vi "Config Voltage.vi"(0 "VISA resource name":refnum<visa-resource-name>, 1 "Element (0: All)":u16(ring) items=["All", "Element 1", "Element 2", "Element 3", "Element 4"], 7 "V Range (8: 2000)":u16(ring)=8 items=["AUTO", "30", "60", "120", "200", "300", "600", "1200", "2000"], 11 "error in (no error)":errorcluster) -> (4 "VISA resource name out":refnum<visa-resource-name>, 15 "error out":errorcluster)   [LabVIEW 2013, in "Yokogawa PZ4000.lvlib"]
doc: "This VI sends the Voltage Configure command to the PZ4000 series.\nConfigure Control Functions are Selects the Voltage Mode, Voltage Range and Element."
uses:
  <instrlib>/Yokogawa PZ4000/Yokogawa PZ4000.lvlib
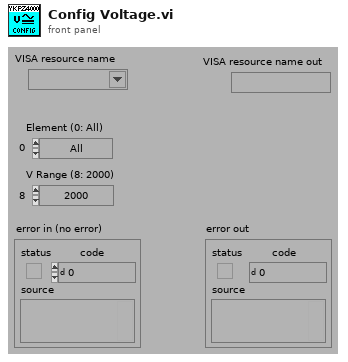
[diagram p1: front panel]
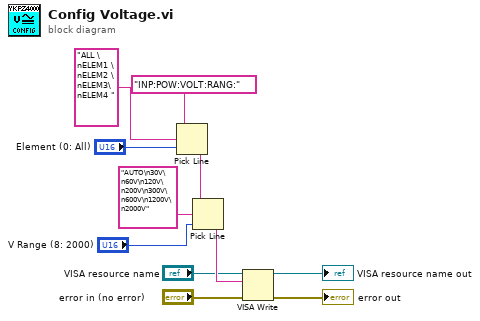
[diagram p0: block diagram]
diagram:
  n1 = Pick Line(string ("")="INP:POW:VOLT:RANG:", multi-line string="ALL \nELEM1 \nELEM2 \nELEM3\nELEM4 ", line index="Element (0: All)") -> (output string=w4:string)
  n2 = Pick Line(string ("")=w4, multi-line string="AUTO\n30V\n60V\n120V\n200V\n300V\n600V\n1200V\n2000V", line index="V Range (8: 2000)") -> (output string=w9:string)
  n3 = VISA Write(VISA resource name="VISA resource name", write buffer=w9, error in (no error)="error in (no error)") -> (VISA resource name out=→"VISA resource name out":refnum<visa-resource-name>, error out=→"error out":errorcluster)  [unwired: 1 out]
